vi "Shake Tray Impl.vi"(8 "error in (no error)":errorcluster, 10 "Time (s)":dbl=1.0, 11 "Alltesta Autosampler in":refnum<class "Alltesta Autosampler.lvclass">) -> (0 "error out":errorcluster, 3 "Alltesta Autosampler out":refnum<class "Alltesta Autosampler.lvclass">)   [LabVIEW 2023, in "Alltesta Autosampler.lvlib" / "Alltesta Autosampler.lvclass"]
uses:
  Alltesta Autosampler.lvclass
  Alltesta Autosampler.lvclass/Alltesta Autosampler.ctl
  Alltesta Autosampler.lvlib
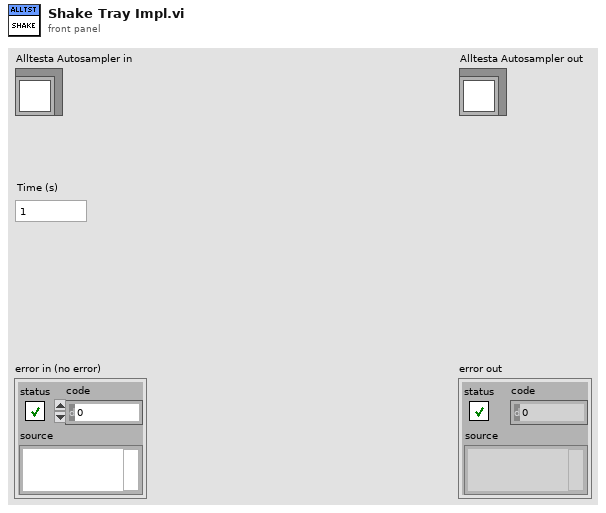
[diagram p1: front panel]
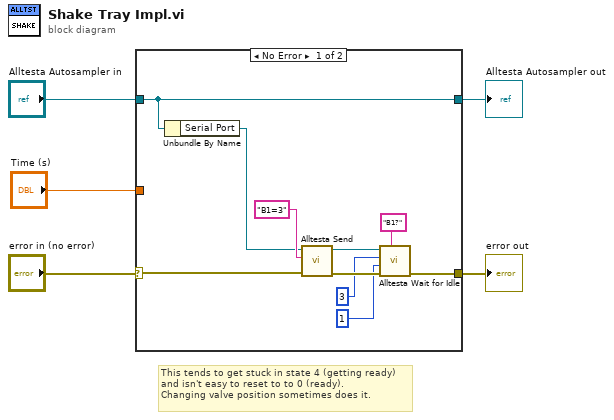
[diagram p0: block diagram]
diagram:
  # "This tends to get stuck in state 4 (getting ready)\nand isn't easy to reset to to 0 (ready).\nChanging valve position sometimes does it."
  n1 = case shown="No Error" "error in (no error)" {
    selector: "error in (no error)" -> [w13 w17]
    tunnel: "Alltesta Autosampler in" -> [w15 w16]
    tunnel: [w15 w16] -> w3
    tunnel: [w6 w17] -> w2
    tunnel: "Time (s)" -> [_ _]
    frame No Error {
      n2 = Unbundle By Name(w15) -> ("Serial Port"=w12:refnum<visa-resource-name>)
      n3 = call "Alltesta Send.vi"("error in (no error)"=w13, "Command"="B1=3", "Serial Port in"=w12) -> ("error out"=w11:errorcluster, "Serial Port out"=w10:refnum<visa-resource-name>)  [unwired: 6 in, 1 out]
      n4 = call "Alltesta Wait for Idle.vi"("Poll Command"="B1?", "error in (no error)"=w11, "Lower Bound"=1, "Upper Bound"=3, "Serial Port in"=w10) -> ("error out"=w6:errorcluster)  [unwired: 5 in, 1 out]
    }
    frame Error {
    }
  }
  "error out" <- w2
  "Alltesta Autosampler out" <- w3
